vi "target.vi"() -> ()   [LabVIEW 2020]
uses:
  <vilib>/rvi/interface/RandomDataEmulation/niFpgaRandomDataHandleErrors.vi
  <vilib>/rvi/DataTransferAndStorage/Container/XNode/niFpgaContainer.xnode
  <vilib>/rvi/interface/RandomDataEmulation/nirviRandomDataFpgaReadWriteTemplate.vi
panel:
  out "tick count":u32
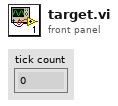
[diagram p1: front panel]
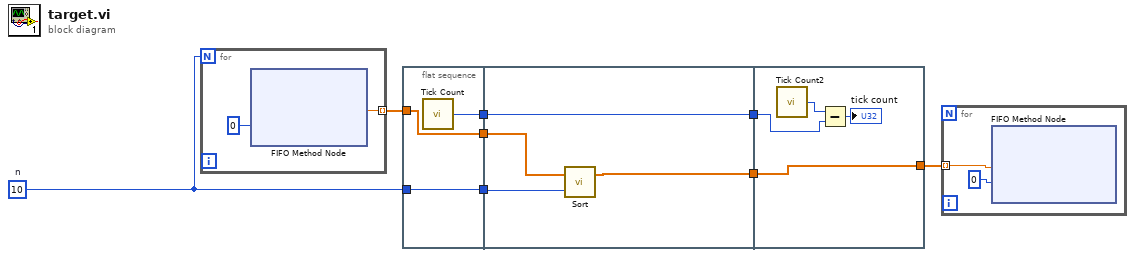
[diagram p0: block diagram]
diagram:
  w3 = 10  # n
  n1 = for {
    N: w3 -> [_]
    tunnel: [w10] -> w8 mode=indexing
    n2 = xnode ("FIFO Method Node")("Timeout"=0) -> ("Element"=w10:sgl)  [unwired: 1 in, 2 out]
  }
  n3 = flat-sequence {
    tunnel: w3 -> [w12]
    tunnel: w8 -> [w13]
    tunnel: [w13] -> w7
    tunnel: [w12] -> w6
    tunnel: [w11] -> w5
    tunnel: w7 -> [w16]
    tunnel: w6 -> [w15]
    tunnel: w5 -> [w17]
    tunnel: [w17] -> w4
    tunnel: [w14] -> w2
    tunnel: w4 -> [w20]
    tunnel: w2 -> [w18]
    tunnel: [w18] -> w1
    frame #0 {
      n4 = call "Tick Count"() -> ("Tick Count(Ticks)"=w11:u32)
    }
    frame #1 {
      n5 = call <vilib>:"Sort.vi"("n"=w15, "Real"=w16) -> ("Sorted A"=w14:sgl[])  [unwired: 1 in]
    }
    frame #2 {
      n6 = call "Tick Count2"() -> ("Tick Count(Ticks)"=w21:u32)
      n7 = Subtract(x=w21, y=w20) -> (x-y=→"tick count":u32)
    }
  }
  n8 = for {
    tunnel: w1 -> [w22] mode=indexing
    n9 = xnode ("FIFO Method Node")("Element"=w22, "Timeout"=0) -> ()  [unwired: 1 in, 2 out]
  }
